vi "Main.vi"() -> ()   [LabVIEW 2023]
panel:
  in  "module path":path=path "C:/TechnologyLab/NI-2010/Drivers/Python Example/Python Scripts/Add Example.py"
  out "Output":dbl
  in  "Input2":dbl=3.0
  in  "Input1":dbl=2.0
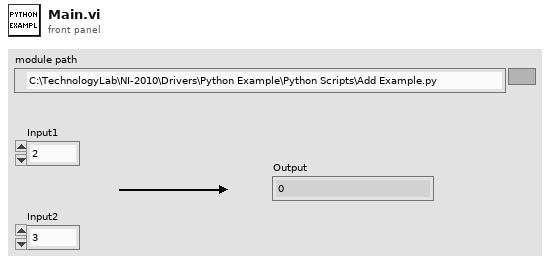
[diagram p1: front panel]
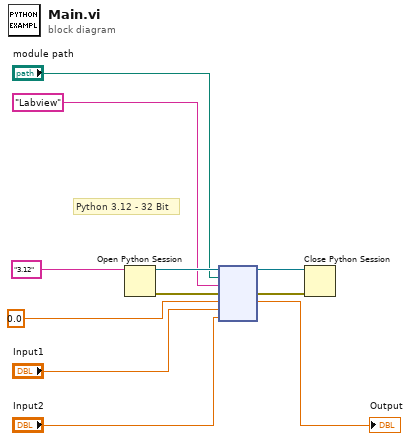
[diagram p0: block diagram]
diagram:
  # "Python 3.12 - 32 Bit"
  n1 = Open Python Session(python version="3.12" ("Python version")) -> (session out=w9:refnum<k35>, error out=w11:errorcluster)  [unwired: 2 in]
  n2 = node(w9, "module path", "Labview" ("function name"), w11, 0.0, "Input1", "Input2") -> (w8:refnum<k35>, w10:errorcluster, →"Output":dbl)  [unwired: 2 in, 2 out]
  n3 = Close Python Session(session in=w8, error in=w10) -> ()  [unwired: 1 out]
